vi "BallShear.vi"() -> ()   [LabVIEW 2013]
panel:
  out "Ready":bool
  in  "Power":bool
  in  "Options":enum32{"Shear", "Results", "Settings"}(tab)
  in  "Ball Selection":i32[](listbox)
  out "OK":bool
  out "Package":picture
  out "Status":string
  in  "Proceed":bool
  out "Step":dbl
  in  "Preceed":bool
  in  "Remove Package":bool
  out "Total Steps":dbl
  in  "Check":bool caption="Ball and Speed Selection"
  out "Array":cluster{"Waveform Chart":dbl[]}[](array[cluster]) caption="Array of clusters, each containing one waveform chart"
  out "Default Image":path
  out "Package Image":path
  out "Analyzed Image":path
  out "Force Reading":path
  out "RCoord":path
  out "VCoord":path
  out "Coord_Conversion":path
  out "Ball_Detection":path
  out "Livefeed":path
  out "Displayed Image":path=path "C:/Users/nsliwa/Documents/GitHub/Ball_Shear/Images/default.jpg"
  out "Coordinates":dbl[][](array[numeric])
  out "Ball IDs":string[](array[string])
  in  "Empty Array":dbl[][](array[numeric])
  out "Selected Indices":dbl[](array[numeric])
  out "Selected \nCoordinates":dbl[][](array[numeric])
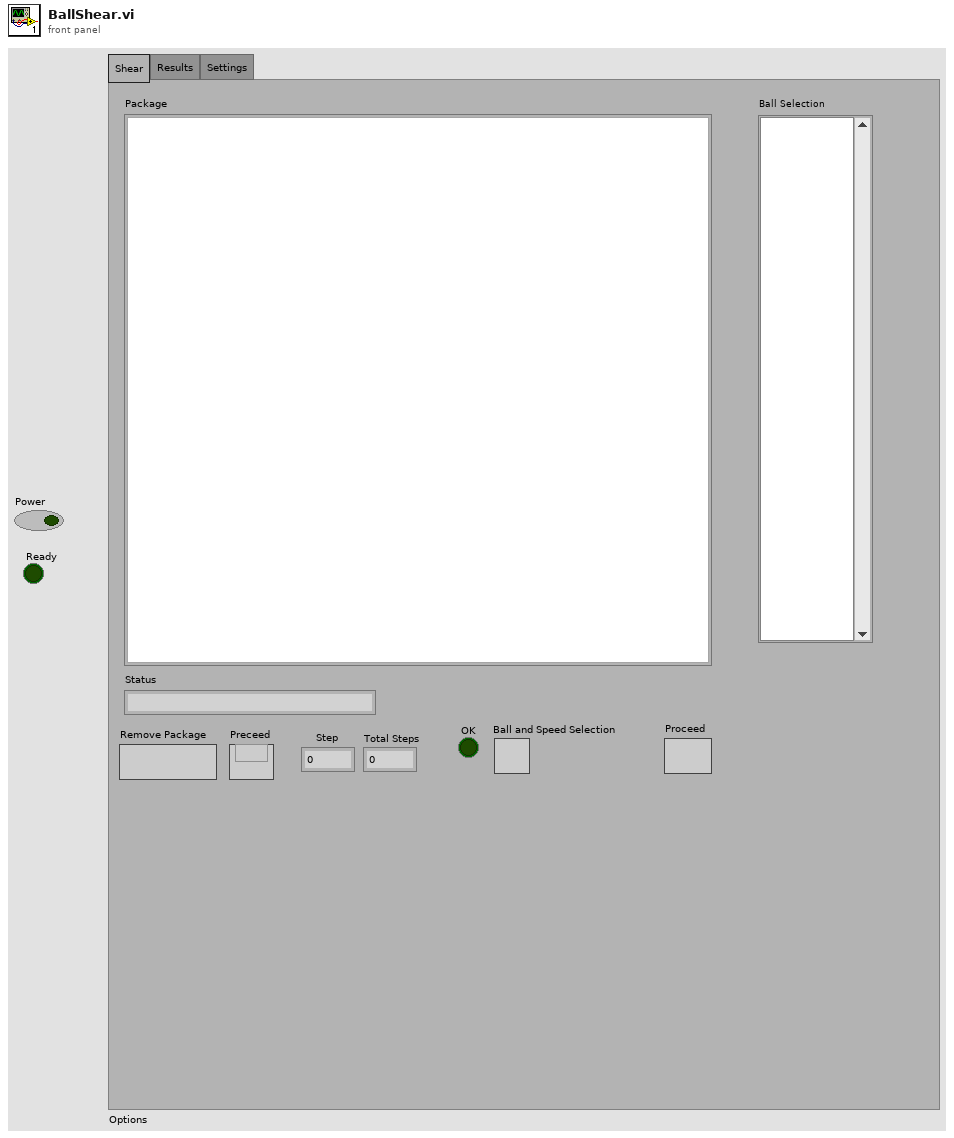
[diagram p1: front panel]
types:
  T1 = typedef "imagedata.ctl" = cluster{"image type":i32, "image depth":i32, "image":u8[], "mask":u8[], "colors":u32[], "Rectangle":cluster{"left":i16, "top":i16, "right":i16, "bottom":i16}}
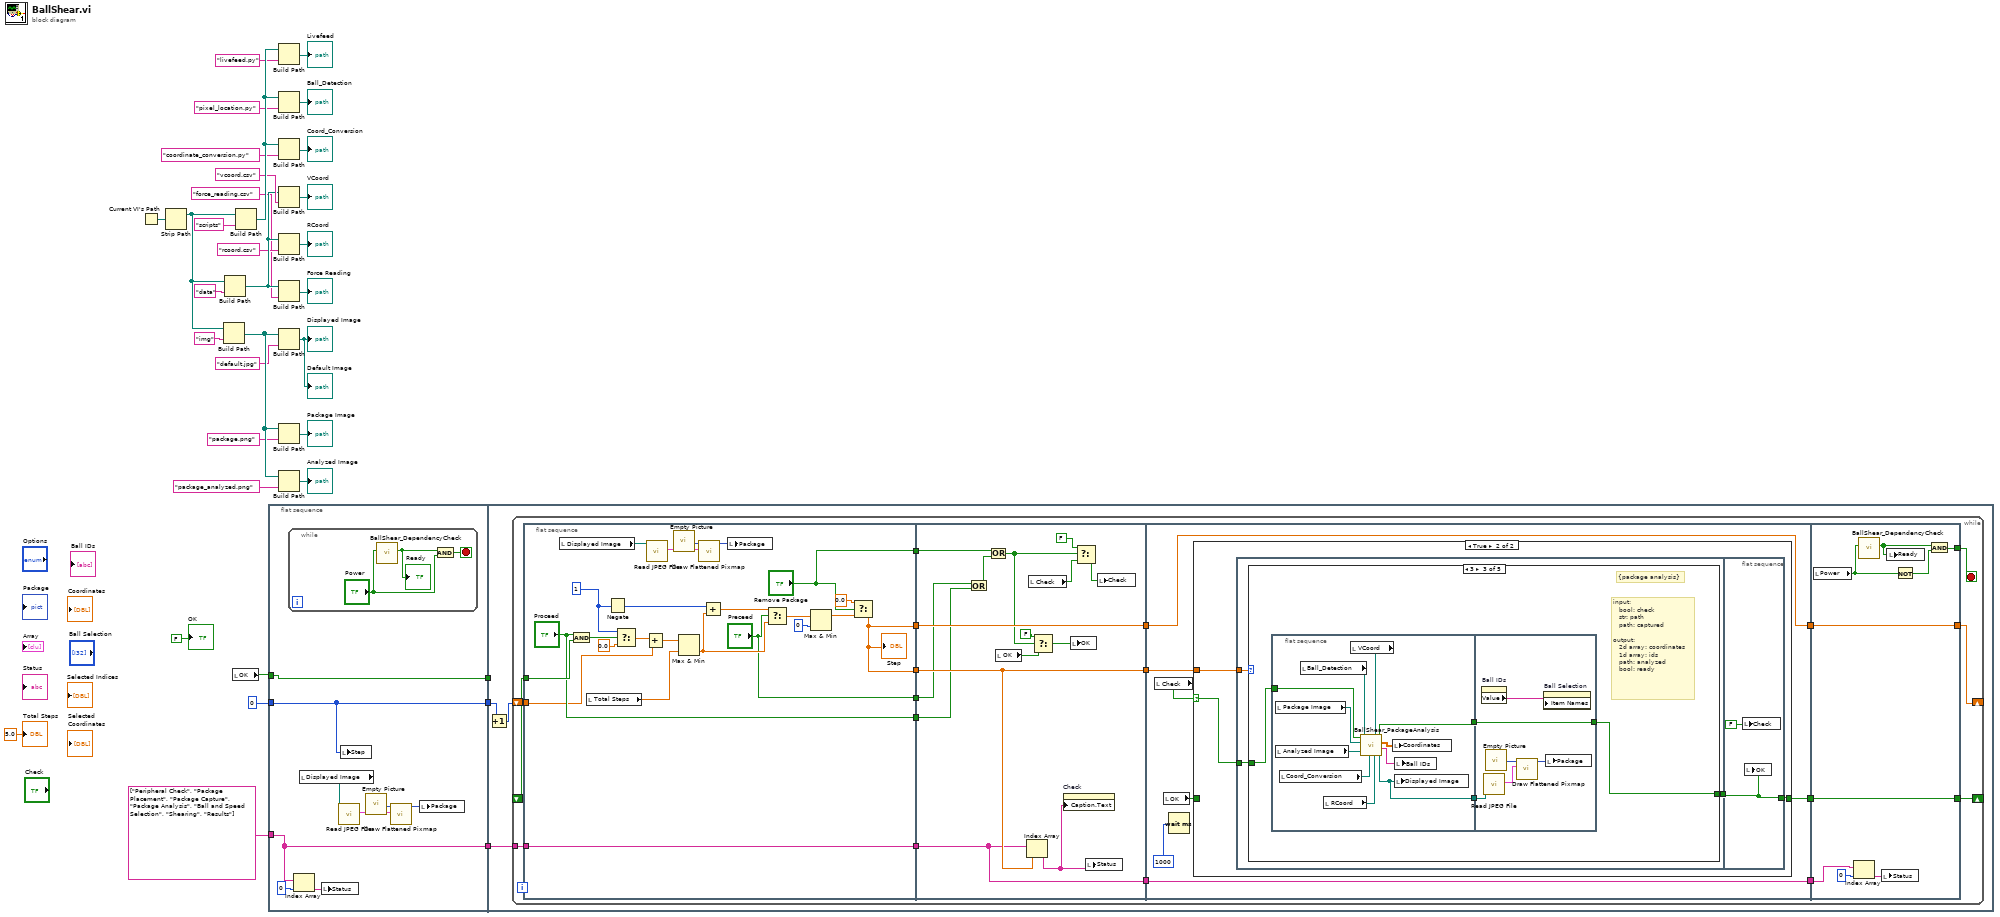
[diagram p0: block diagram]
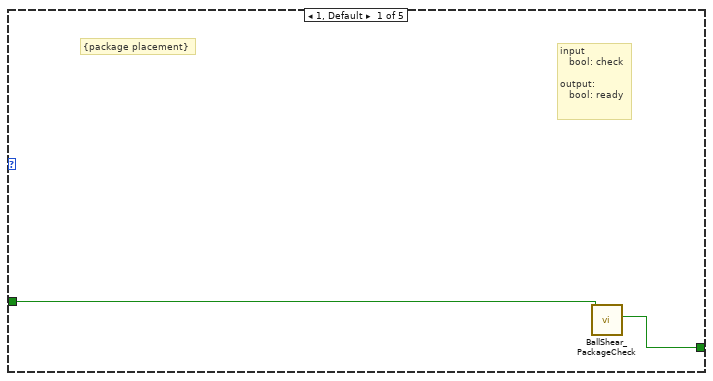
[diagram p3: hidden frame]
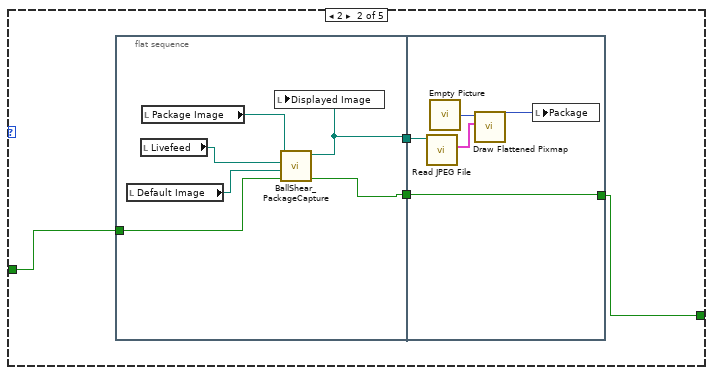
[diagram p4: hidden frame]
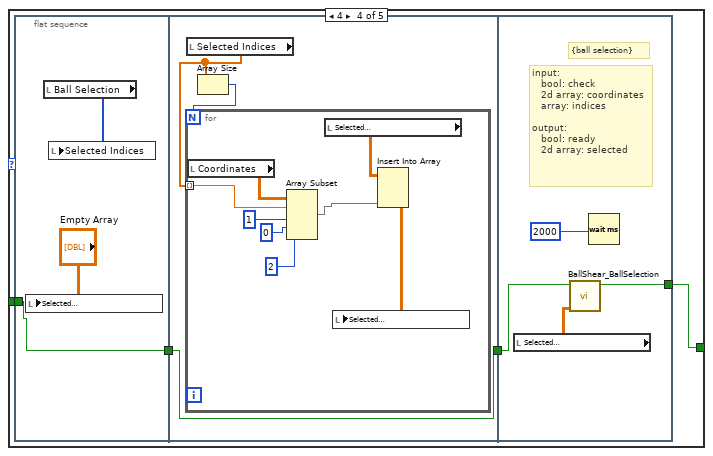
[diagram p5: hidden frame]
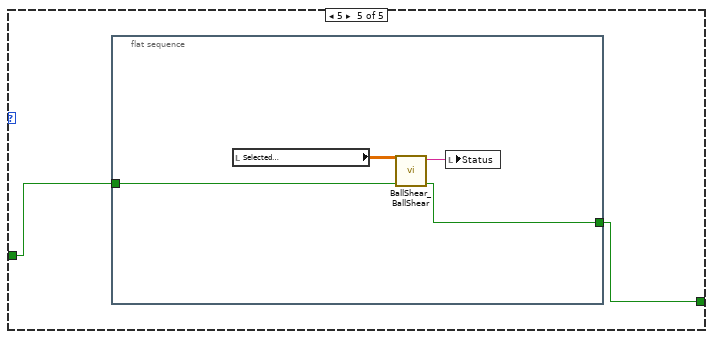
[diagram p6: hidden frame]
diagram:
  n1 = Current VI's Path() -> (path=w34:path)
  n2 = Strip Path(path=w34) -> (stripped path=w32:path)  [unwired: 1 out]
  n3 = Build Path(base path=w32, name or relative path="img") -> (appended path=w29:path)
  n4 = Build Path(base path=w32, name or relative path="data") -> (appended path=w23:path)
  n5 = local read "OK"() -> (w2:bool)
  n6 = Build Path(base path=w32, name or relative path="scripts") -> (appended path=w28:path)
  n7 = flat-sequence {
    tunnel: string[] ["Peripheral Check", "Package Placement", "Package Capture", "Package Analysis", "Ball and Speed Selection", "Shearing", "Results"] -> [w41]
    tunnel: [w41] -> w7
    tunnel: w2 -> [w40]
    tunnel: [w40] -> w6
    tunnel: [w39] -> w5
    tunnel: 0 -> [w39]
    tunnel: w7 -> [w49]
    tunnel: w6 -> [_]
    tunnel: w5 -> [w48]
    frame #0 {
      n8 = while {
        stop <- w46 stop-if-true
        n9 = call "BallShear_DependencyCheck.vi"("Power"="Power") -> ("Ready"=w45:bool)  [unwired: 10 in]
        "Ready" <- w45
        n10 = And(x=w45, y="Power") -> (x .and. y?=w46:bool)
      }
      n11 = Index Array(array=w41, index=0) -> (element=w42:string)
      n12 = local read "Displayed Image"() -> (w35:path)
      n13 = local write "Status"(w42) -> ()
      n14 = call <vilib>:"Read JPEG File.vi"("path to JPEG file"=w35) -> ("image data"=w36:T1)  [unwired: 8 in, 2 out]
      n15 = local write "Step"(w39) -> ()
      n16 = call "Empty Picture"() -> ("empty picture"=w37:picture)
      n17 = call <vilib>:"Draw Flattened Pixmap.vi"("image data"=w36, "picture"=w37) -> ("new picture"=w38:picture)  [unwired: 7 in]
      n18 = local write "Package"(w38) -> ()
    }
    frame #1 {
      n19 = Increment(x=w48) -> (x+1=w47:i32)
      n20 = while {
        tunnel: w49 -> [w65]
        shift-right: [w52] -> _
        shift-left: _ -> [w62]
        shift-right: [w57] -> _
        shift-left: w47 -> [w60]
        stop <- w67 stop-if-true
        n21 = flat-sequence {
          tunnel: [w74] -> w66
          tunnel: w65 -> [w74]
          tunnel: [w72] -> w64
          tunnel: w62 -> [w73]
          tunnel: [w72] -> w61
          tunnel: w60 -> [w68]
          tunnel: ["Proceed"] -> w56
          tunnel: ["Preceed"] -> w55
          tunnel: ["Remove Package"] -> w54
          tunnel: w66 -> [w96]
          tunnel: w64 -> [w106]
          tunnel: [w106] -> w63
          tunnel: w61 -> [w102]
          tunnel: [w102] -> w59
          tunnel: w56 -> [w99]
          tunnel: w55 -> [w101]
          tunnel: w54 -> [w100]
          tunnel: [w96] -> w51
          tunnel: w63 -> [w112]
          tunnel: w59 -> [w111]
          tunnel: [w111] -> w58
          tunnel: [w109] -> w53
          tunnel: w51 -> [w108]
          tunnel: [w108] -> w50
          tunnel: [w195] -> w67
          tunnel: [w194] -> w57
          tunnel: w58 -> [w194]
          tunnel: w53 -> [w193]
          tunnel: [w193] -> w52
          tunnel: w50 -> [w190]
          frame #0 {
            w75 = 1
            n22 = local read "Displayed Image"() -> (w91:path)
            n23 = And(x="Proceed", y=w73) -> (x .and. y?=w76:bool)
            n24 = local read "Total Steps"() -> (w78:dbl)
            n25 = Negate(x=w75) -> (-x=w86:i32)
            n26 = Select(t=w75, s=w76, f=0.0) -> (s? t:f=w85:dbl)
            n27 = Add(x=w85, y=w68) -> (x+y=w83:dbl)
            n28 = call <vilib>:"Read JPEG File.vi"("path to JPEG file"=w91) -> ("image data"=w90:T1)  [unwired: 8 in, 2 out]
            n29 = call "Empty Picture"() -> ("empty picture"=w89:picture)
            n30 = Max & Min(x=w83, y=w78) -> (min(x,y)=w82:dbl)  [unwired: 1 out]
            n31 = call <vilib>:"Draw Flattened Pixmap.vi"("image data"=w90, "picture"=w89) -> ("new picture"=w88:picture)  [unwired: 7 in]
            n32 = Add(x=w86, y=w82) -> (x+y=w87:dbl)
            n33 = local write "Package"(w88) -> ()
            n34 = Select(t=w87, s="Preceed", f=w82) -> (s? t:f=w81:dbl)
            n35 = Max & Min(x=w81, y=i16 0) -> (max(x,y)=w80:dbl)  [unwired: 1 out]
            n36 = Select(t=0.0, s="Remove Package", f=w80) -> (s? t:f=w72:dbl)
            "Step" <- w72
          }
          frame #1 {
            n37 = Or(x=w101, y=w99) -> (x .or. y?=w103:bool)
            n38 = Or(x=w100, y=w103) -> (x .or. y?=w95:bool)
            n39 = local read "OK"() -> (w93:bool)
            n40 = Index Array(array=w96, index=w106) -> (element=w97:string)
            n41 = local read "Check"() -> (w105:bool)
            n42 = Select(t=FALSE, s=w95, f=w93) -> (s? t:f=w94:bool)
            n43 = property on="Check" class="Bool (strict)"("Caption.Text"=w97) -> ()  [unwired: 2 in, 2 out]
            n44 = local write "OK"(w94) -> ()
            n45 = Select(t=FALSE, s=w95, f=w105) -> (s? t:f=w98:bool)
            n46 = local write "Status"(w97) -> ()
            n47 = local write "Check"(w98) -> ()
          }
          frame #2 {
            n48 = local read "Check"() -> (w113:bool)
            n49 = local read "OK"() -> (w110:bool)
            n50 = Wait (ms)(milliseconds to wait=u32 1000) -> ()  [unwired: 1 out]
            n51 = case shown="True" w113 {
              selector: w113 -> [_ w115]
              tunnel: w112 -> [_ w118]
              tunnel: [w114 w117] -> w109
              tunnel: w110 -> [w114 _]
              frame False {
              }
              frame True {
                n52 = flat-sequence {
                  tunnel: w118 -> [w121]
                  tunnel: [w120] -> w116
                  tunnel: w115 -> [w119]
                  tunnel: [w188] -> w117
                  tunnel: w116 -> [w188]
                  frame #0 {
                    n53 = case shown="3" w121 {
                      tunnel: [w123 w125 w140 w163 w182] -> w120
                      tunnel: w119 -> [w122 w124 w139 w161 w183]
                      frame 1, Default {
                        # "{package placement}"
                        # "input\n   bool: check\n\noutput:\n   bool: ready"
                        n54 = call "BallShear_PackageCheck.vi"("Check"=w122) -> ("Ready"=w123:bool)  [unwired: 10 in]
                      }
                      frame 2 {
                        n55 = flat-sequence {
                          tunnel: [w129] -> w127
                          tunnel: [w133] -> w126
                          tunnel: w124 -> [w128]
                          tunnel: w127 -> [w134]
                          tunnel: w126 -> [w136]
                          tunnel: [w134] -> w125
                          frame #0 {
                            n56 = local read "Default Image"() -> (w130:path)
                            n57 = local read "Livefeed"() -> (w131:path)
                            n58 = local read "Package Image"() -> (w132:path)
                            n59 = call "BallShear_PackageCapture.vi"("Capture"=w128, "Default Image Path"=w130, "Python Script Path"=w131, "Target Image Path"=w132) -> ("Success"=w129:bool, "Actual Image Path"=w133:path)  [unwired: 6 in]
                            n60 = local write "Displayed Image"(w133) -> ()
                          }
                          frame #1 {
                            n61 = call <vilib>:"Read JPEG File.vi"("path to JPEG file"=w136) -> ("image data"=w138:T1)  [unwired: 8 in, 2 out]
                            n62 = call "Empty Picture"() -> ("empty picture"=w137:picture)
                            n63 = call <vilib>:"Draw Flattened Pixmap.vi"("image data"=w138, "picture"=w137) -> ("new picture"=w135:picture)  [unwired: 7 in]
                            n64 = local write "Package"(w135) -> ()
                          }
                        }
                      }
                      frame 3 {
                        # "input:\n   bool: check\n   str: path\n   path: captured\n\noutput:\n   2d array: coordinates\n   1d array: ids\n   path: analyzed\n   bool: ready"
                        # "{package analysis}"
                        n65 = flat-sequence {
                          tunnel: [w151] -> w142
                          tunnel: [w150] -> w141
                          tunnel: w139 -> [w143]
                          tunnel: w142 -> [w159]
                          tunnel: w141 -> [w155]
                          tunnel: [w159] -> w140
                          frame #0 {
                            n66 = local read "Package Image"() -> (w147:path)
                            n67 = local read "Analyzed Image"() -> (w146:path)
                            n68 = local read "Coord_Conversion"() -> (w145:path)
                            n69 = local read "Ball_Detection"() -> (w148:path)
                            n70 = local read "RCoord"() -> (w144:path)
                            n71 = local read "VCoord"() -> (w149:path)
                            n72 = call "BallShear_PackageAnalysis.vi"("Real Coordinates"=w144, "Virtual Coordinates"=w149, "Coord Conversion Script"=w145, "Package Analysis Script"=w148, "Analyzed Package Path"=w146, "Original Package Path"=w147, "Analyze"=w143) -> ("Displayed Path"=w150:path, "IDs"=w152:string[], "Coordinates"=w153:dbl[][], "Success"=w151:bool)  [unwired: 1 in]
                            n73 = local write "Coordinates"(w153) -> ()
                            n74 = local write "Displayed Image"(w150) -> ()
                            n75 = local write "Ball IDs"(w152) -> ()
                          }
                          frame #1 {
                            n76 = property on="Ball IDs" class="Arr (strict)"() -> ("Value"=w154:string[])  [unwired: 2 in, 2 out]
                            n77 = call <vilib>:"Read JPEG File.vi"("path to JPEG file"=w155) -> ("image data"=w158:T1)  [unwired: 8 in, 2 out]
                            n78 = call "Empty Picture"() -> ("empty picture"=w157:picture)
                            n79 = call <vilib>:"Draw Flattened Pixmap.vi"("image data"=w158, "picture"=w157) -> ("new picture"=w156:picture)  [unwired: 7 in]
                            n80 = property on="Ball Selection" class="LstBox (strict)"("Item Names"=w154) -> ()  [unwired: 2 in, 2 out]
                            n81 = local write "Package"(w156) -> ()
                          }
                        }
                      }
                      frame 4 {
                        n82 = flat-sequence {
                          tunnel: [w164] -> w162
                          tunnel: w161 -> [w164]
                          tunnel: w162 -> [w167]
                          tunnel: [w167] -> w160
                          tunnel: [w179] -> w163
                          tunnel: w160 -> [w178]
                          frame #0 {
                            n83 = local write "Selected \nCoordinates"("Empty Array") -> ()
                            n84 = local read "Ball Selection"() -> (w166:i32[])
                            n85 = local write "Selected Indices"(w166) -> ()
                          }
                          frame #1 {
                            n86 = local read "Selected Indices"() -> (w168:dbl[])
                            n87 = Array Size(array=w168) -> (size(s)=w169:i32)
                            n88 = for {
                              N: w169 -> [_]
                              tunnel: w168 -> [w172] mode=indexing
                              n89 = local read "Coordinates"() -> (w176:dbl[][])
                              n90 = Array Subset(array=w176, index (row)=w172, length (row)=1 ("length"), index (col)=0 ("index"), length (col)=2 ("length")) -> (w173:dbl[][])
                              n91 = local read "Selected \nCoordinates"() -> (w177:dbl[][])
                              n92 = Insert Into Array(array=w177, new element=w173) -> (w170:dbl[][])  [unwired: 2 in]
                              n93 = local write "Selected \nCoordinates"(w170) -> ()
                            }
                          }
                          frame #2 {
                            # "input:\n   bool: check\n   2d array: coordinates\n   array: indices\n\noutput: \n   bool: ready\n   2d array: selected"
                            # "{ball selection}"
                            n94 = local read "Selected \nCoordinates"() -> (w180:dbl[][])
                            n95 = call "BallShear_BallSelection.vi"("Selected Balls"=w180, "Check"=w178) -> ("Ready"=w179:bool)  [unwired: 9 in]
                            n96 = Wait (ms)(milliseconds to wait=u32 2000) -> ()  [unwired: 1 out]
                          }
                        }
                      }
                      frame 5 {
                        n97 = flat-sequence {
                          tunnel: [w184] -> w182
                          tunnel: w183 -> [w185]
                          frame #0 {
                            n98 = local read "Selected \nCoordinates"() -> (w187:dbl[][])
                            n99 = call "BallShear_BallShear.vi"("Check"=w185, "Selected Balls"=w187) -> ("Ready"=w184:bool, "Status"=w186:string)  [unwired: 8 in]
                            n100 = local write "Status"(w186) -> ()
                          }
                        }
                      }
                    }
                  }
                  frame #1 {
                    n101 = local write "Check"(FALSE ("Check")) -> ()
                    n102 = local write "OK"(w188) -> ()
                  }
                }
              }
            }
          }
          frame #3 {
            n103 = local read "Power"() -> (w197:bool)
            n104 = Index Array(array=w190, index=0) -> (element=w192:string)
            n105 = call "BallShear_DependencyCheck.vi"("Power"=w197) -> ("Ready"=w196:bool)  [unwired: 10 in]
            n106 = local write "Status"(w192) -> ()
            n107 = local write "Ready"(w196) -> ()
            n108 = Not(x=w197) -> (.not. x?=w198:bool)
            n109 = And(x=w196, y=w198) -> (x .and. y?=w195:bool)
          }
        }
      }
    }
  }
  n110 = Build Path(base path=w28, name or relative path="livefeed.py") -> (appended path=→"Livefeed":path)
  n111 = Build Path(base path=w28, name or relative path="pixel_location.py") -> (appended path=→"Ball_Detection":path)
  n112 = Build Path(base path=w28, name or relative path="coordinate_conversion.py") -> (appended path=→"Coord_Conversion":path)
  n113 = Build Path(base path=w23, name or relative path="vcoord.csv") -> (appended path=→"VCoord":path)
  n114 = Build Path(base path=w23, name or relative path="rcoord.csv") -> (appended path=→"RCoord":path)
  n115 = Build Path(base path=w23, name or relative path="force_reading.csv") -> (appended path=→"Force Reading":path)
  n116 = Build Path(base path=w29, name or relative path="default.jpg") -> (appended path=→"Displayed Image" →"Default Image":path)
  n117 = Build Path(base path=w29, name or relative path="package.png") -> (appended path=→"Package Image":path)
  n118 = Build Path(base path=w29, name or relative path="package_analyzed.png") -> (appended path=→"Analyzed Image":path)
  "Total Steps" <- 5.0 ("Total Steps")
  "OK" <- FALSE
